vi "publisher_subscriber.vi"() -> ()   [LabVIEW 2014]
uses:
  Map_lib/MapBuilder/Robot_Position.ctl
  <vilib>/Tufts CEEO ROS for LabVIEW Software/ROS/Code/Console/Servers/ServerSubs/TopicDef.ctl
  <vilib>/Tufts CEEO ROS for LabVIEW Software/ROS/Code/SubVIs/_ROSDirection.ctl
panel:
  in  "cmdvel":T1={"msg.x"=1.01, "msg.y"=0.0, "msg.theta"=0.0}
  in  "停止":bool
  in  "发送":bool
  out "错误输出":errorcluster
  out "sensor_msg_cluster":cluster{"voltage":dbl, "motor":i8}
  out "robot_position_cluster":T2
  in  "stop2":bool
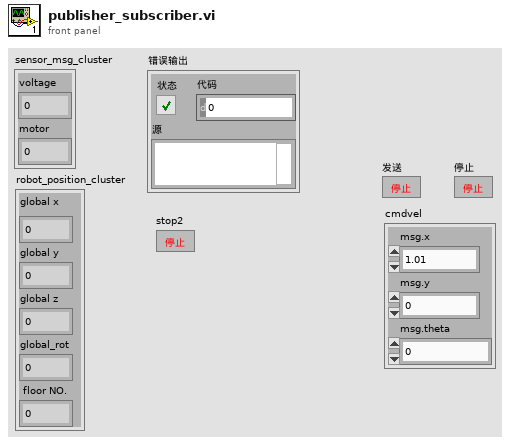
[diagram p1: front panel]
types:
  T1 = cluster{"msg.x":dbl, "msg.y":dbl, "msg.theta":dbl}
  T2 = typedef "Robot_Position.ctl" = cluster{"global x":dbl, "global y":dbl, "global z":dbl, "global_rot":dbl, " floor NO.":dbl}
  T3 = typedef "TopicDef.ctl" = cluster{"Topic":string, "Type":string, "Action":T4, "Update (ms)":u16, "queue size":u16}
  T4 = typedef "_ROSDirection.ctl" = enum16{"Node", "Publisher", "Subscriber", "ServiceClient", "ServiceProvider"}
  T5 = typedef "_ROSControl.ctl" = cluster{"topic port":u16, "Node":string, "topic":string, "type":string, "node port":u16, "error ":errorcluster, "Direction":T4, "Update (ms)":u16, "FIFO size":u16}
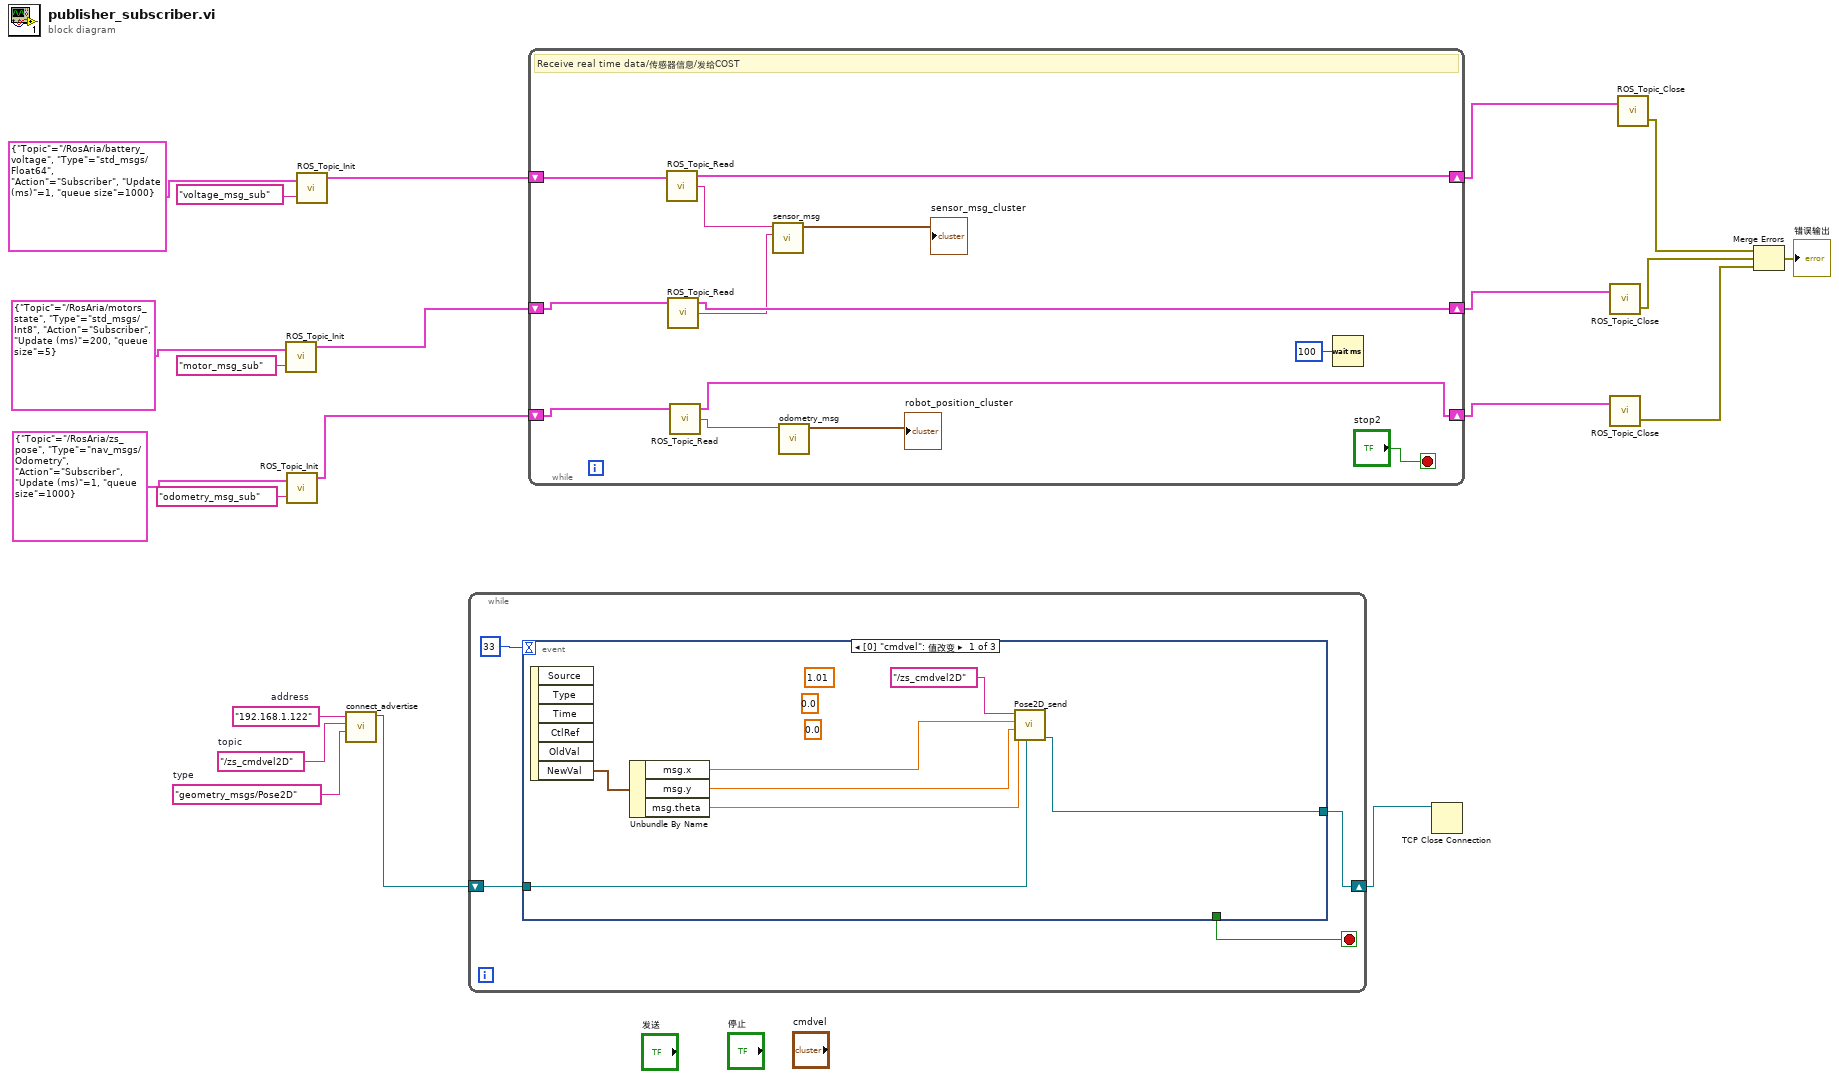
[diagram p0: block diagram]
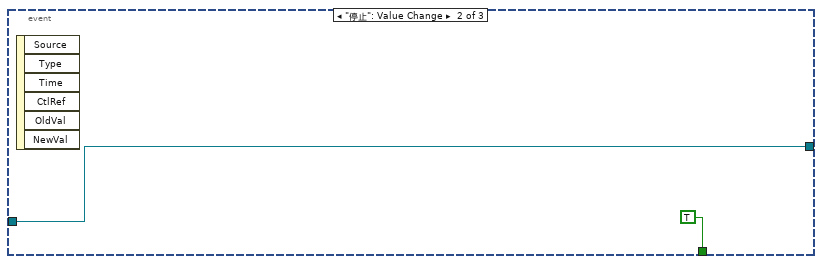
[diagram p2: hidden frame]
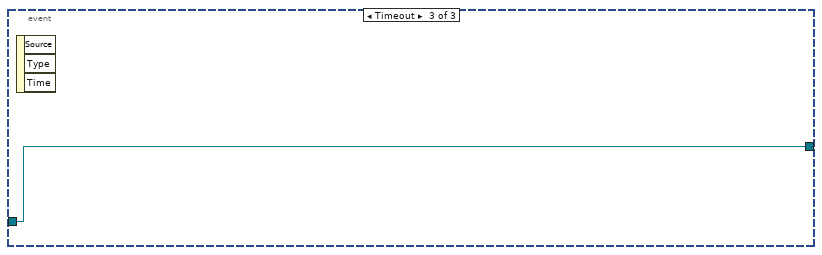
[diagram p3: hidden frame]
diagram:
  w4 = "192.168.1.122"  # address
  w3 = "/zs_cmdvel2D"  # topic
  w1 = "geometry_msgs/Pose2D"  # type
  n1 = call <vilib>:"ROS_Topic_Init.vi"("Definitions"=T3 {"Topic"="/RosAria/motors_state", "Type"="std_msgs/Int8", "Action"=enum."Subscriber", "Update (ms)"=200, "queue size"=5}, "node"="motor_msg_sub") -> ("ROS out"=w15:T5)  [unwired: 1 in, 1 out]
  n2 = call <vilib>:"ROS_Topic_Init.vi"("Definitions"=T3 {"Topic"="/RosAria/zs_pose", "Type"="nav_msgs/Odometry", "Action"=enum."Subscriber", "Update (ms)"=1, "queue size"=1000}, "node"="odometry_msg_sub") -> ("ROS out"=w11:T5)  [unwired: 1 in, 1 out]
  n3 = call <vilib>:"ROS_Topic_Init.vi"("Definitions"=T3 {"Topic"="/RosAria/battery_voltage", "Type"="std_msgs/Float64", "Action"=enum."Subscriber", "Update (ms)"=1, "queue size"=1000}, "node"="voltage_msg_sub") -> ("ROS out"=w17:T5)  [unwired: 1 in, 1 out]
  n4 = call "connect_advertise.vi"("type"=w1, "topic"=w3, "address"=w4) -> ("连接ID输出"=w2:refnum<k5>)  [unwired: 7 in, 1 out]
  n5 = while {
    shift-right: [w23] -> w5
    shift-left: w2 -> [w22]
    stop <- w24 stop-if-true
    n6 = event shown="[0] \"cmdvel\": 值改变" {
      selector: _ -> [_ _ _]
      dyn-events: _ -> [_ _ _]
      timeout: 33 -> [_ _ _]
      tunnel: [_ TRUE _] -> w24
      tunnel: [w26 w33 w35] -> w23
      tunnel: w22 -> [w32 w33 w35]
      event "cmdvel": Value Change {
        (unwired) 0.0 ("msg.z")
        (unwired) 0.0 ("msg.y")
        (unwired) 1.01 ("msg.x")
        n7 = event-data() -> ("NewVal"=w30:T1)  [unwired: 1 in, 5 out]
        n8 = Unbundle By Name(w30) -> ("msg.x"=w29:dbl, "msg.y"=w28:dbl, "msg.theta"=w27:dbl)
        n9 = call "Pose2D_send.vi"("连接ID"=w32, "msg.theta"=w27, "msg.y"=w28, "msg.x"=w29, "topic"="/zs_cmdvel2D") -> ("连接ID输出"=w26:refnum<k5>)  [unwired: 6 in]
      }
      event "停止": Value Change {
        n10 = event-data() -> ()  [unwired: 1 in, 6 out]
      }
      event Timeout {
        n11 = event-data() -> ()  [unwired: 1 in, 3 out]
      }
    }
  }
  n12 = while {
    shift-right: [w46] -> w16
    shift-left: w17 -> [w47]
    shift-right: [w44] -> w14
    shift-left: w15 -> [w45]
    shift-right: [w42] -> w10
    shift-left: w11 -> [w43]
    stop <- "stop2" stop-if-true
    # "Receive real time data/传感器信息/发给COST"
    n13 = call <vilib>:"ROS_Topic_Read.vi"("ROS in"=w47) -> ("Reply"=w41:string, "ROS out"=w46:T5)  [unwired: 2 in, 1 out]
    n14 = call <vilib>:"ROS_Topic_Read.vi"("ROS in"=w45) -> ("Reply"=w40:string, "ROS out"=w44:T5)  [unwired: 2 in, 1 out]
    n15 = call <vilib>:"ROS_Topic_Read.vi"("ROS in"=w43) -> ("Reply"=w39:string, "ROS out"=w42:T5)  [unwired: 2 in, 1 out]
    n16 = call "sensor_msg.vi"("motor_msg in"=w40, "voltage_msg in"=w41) -> ("sensor_msg_cluster"=→"sensor_msg_cluster":cluster{"voltage":dbl, "motor":i8})  [unwired: 9 in]
    n17 = call "odometry_msg.vi"("odometry_msg in"=w39) -> ("robot_position_cluster"=→"robot_position_cluster":T2)  [unwired: 9 in, 1 out]
    n18 = Wait (ms)(milliseconds to wait=u32 100 ("等待时间（毫秒）")) -> ()  [unwired: 1 out]
  }
  n19 = TCP Close Connection(connection ID=w5) -> ()  [unwired: 2 in, 2 out]
  n20 = call <vilib>:"ROS_Topic_Close.vi"("ROS in"=w14) -> ("error out"=w8:errorcluster)  [unwired: 3 in]
  n21 = call <vilib>:"ROS_Topic_Close.vi"("ROS in"=w10) -> ("error out"=w7:errorcluster)  [unwired: 3 in]
  n22 = call <vilib>:"ROS_Topic_Close.vi"("ROS in"=w16) -> ("error out"=w9:errorcluster)  [unwired: 3 in]
  n23 = Merge Errors(w9, w8, w7) -> (→"错误输出":errorcluster)
